vi "PressureGauge.vi"(4 "Error In":errorcluster, 7 "Command":string) -> (0 "Error Out":errorcluster, 3 "Response":string)   [LabVIEW 2018]
uses:
  MOKO_LabViewLibrary/MokoLowLevel/MokoLowLovelControl/MLLC_Mode.ctl
  data/PressureGaugeInfo.ctl
panel:
  in  "PRESSURESTORE":string="PRESSURESTORE"
  in  "Error Code":i32=5475
  in  "UtilitySettings":T2={"Permanent data"={"Информация об образце"={"Тип"="Манометр", "Владелец"="Компания \"MOKO\"", "Номер клейма"="111222", "Пределы допускаемой погрешности "=0.05, "Производственный № прибора"="111222333", "Наименование СИ"="Манометр"}, "Информация о поверке"={"Место проведения поверки"="Планета земля", "Поверку провел"="Johnny Respect", "Номер заказа"="1", "Номер рабочего места"="1", "ДД"=21.0, "ММ"="Январь", "ГГГГ"=2022.0, "№ протокола"="G-111111", "№ манометра"=5555.0}, "Характеристики манометра"={"Максимум шкалы"=10.0, "1-ая точка"=2.0, "Единица измерения"="МПа", "Цена деления"=2.0, "Класс точности"="0,4", "Минимум шкалы"=2.0, "Количество точек"=0.0}, "Условия поверки"={"Температура воздуха"=22.0, "Влажность воздуха"=60.0, "Давление"=750.0}, "Драйвер"="Simulation", "Поверяемая точка"=0.0}, "Saved Data"=variant(cluster{"Информация об образце":cluster{"Тип":string, "Владелец":string, "Номер клейма":string, "Пределы допускаемой погрешности ":dbl, "Производственный № прибора":string, "Наименование СИ":string}, "Информация о поверке":cluster{"Место проведения поверки":string, "Поверку провел":string, "Номер заказа":string, "Номер рабочего места":string, "ДД":dbl, "ММ":string, "ГГГГ":dbl, "№ протокола":string, "№ манометра":dbl}, "Характеристики манометра":cluster{"Максимум шкалы":dbl, "1-ая точка":dbl, "Единица измерения":string, "Цена деления":dbl, "Класс точности":string, "Минимум шкалы":dbl, "Количество точек":dbl}, "Условия поверки":cluster{"Температура воздуха":dbl, "Влажность воздуха":dbl, "Давление":dbl}, "Драйвер":string, "Поверяемая точка":dbl} {"Информация об образце"={"Тип"="Манометр", "Владелец"="Компания \"MOKO\"", "Номер клейма"="111222333", "Пределы допускаемой погрешности "=0.05, "Производственный № прибора"="111222333", "Наименование СИ"="Манометр"}, "Информация о поверке"={"Место проведения поверки"="Планета земля", "Поверку провел"="Johnny Respect", "Номер заказа"="1", "Номер рабочего места"="1", "ДД"=21.0, "ММ"="Январь", "ГГГГ"=2022.0, "№ протокола"="G-111111", "№ манометра"=1123123.0}, "Характеристики манометра"={"Максимум шкалы"=10.0, "1-ая точка"=2.0, "Единица измерения"="МПа", "Цена деления"=2.0, "Класс точности"="0,4", "Минимум шкалы"=2.0, "Количество точек"=0.0}, "Условия поверки"={"Температура воздуха"=22.0, "Влажность воздуха"=60.0, "Давление"=750.0}, "Драйвер"="Simulation", "Поверяемая точка"=0.0}), "waittime"=30000.0, "BAD"=0.0, "Defect"=FALSE}
  in  "Mode":T3=enum."Check"
  # "PressureGauge"
  # "Default Settings"
  # "Temporary data"
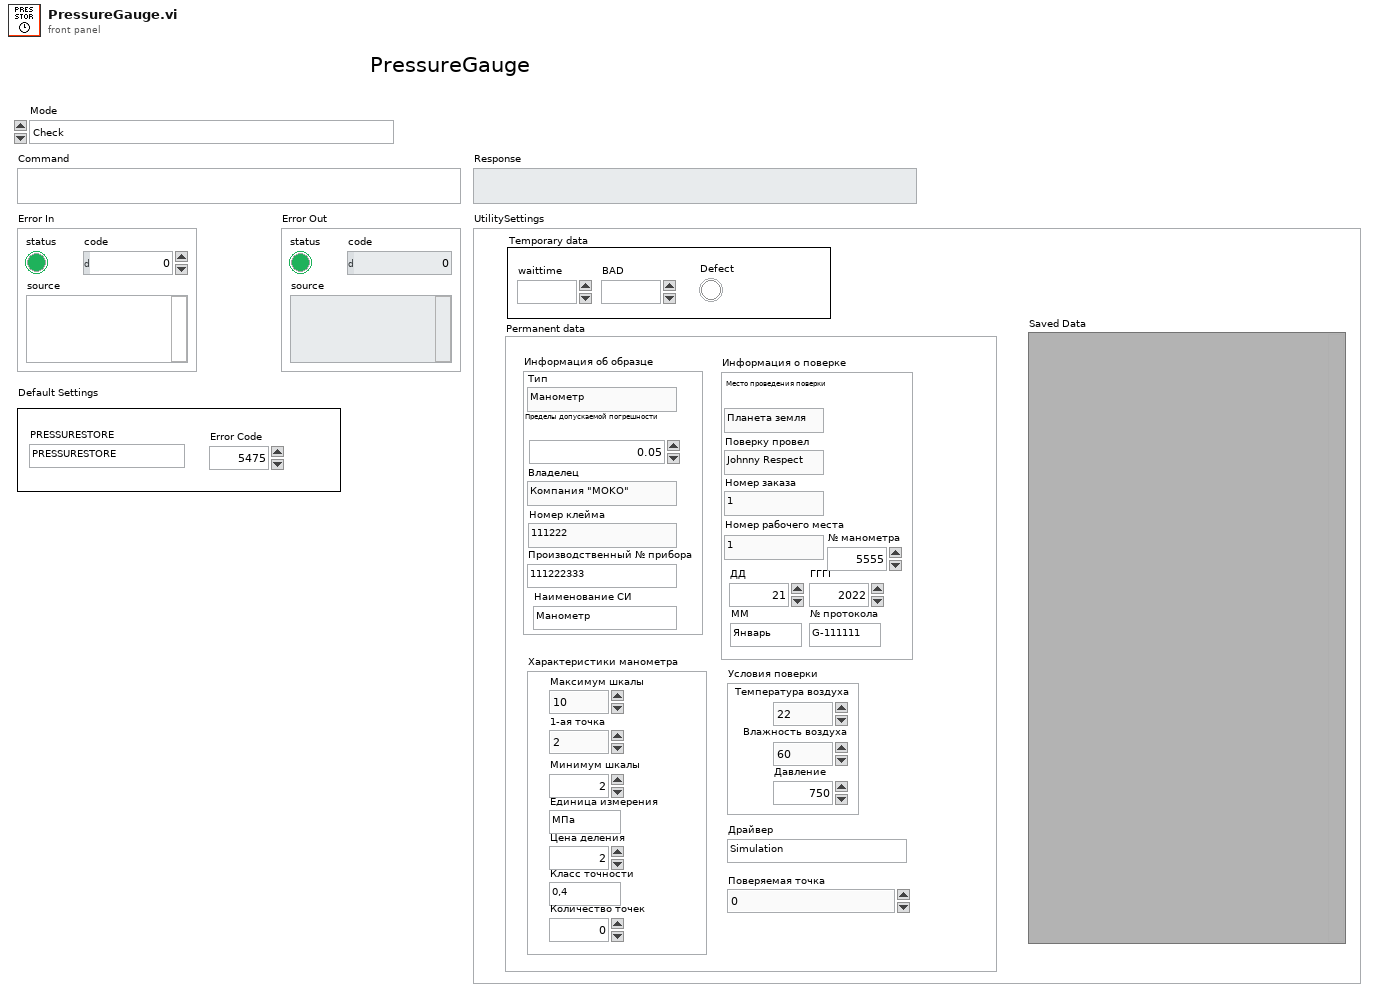
[diagram p1: front panel]
types:
  T1 = typedef "PressureGaugeInfo.ctl" = cluster{"Информация об образце":cluster{"Тип":string, "Владелец":string, "Номер клейма":string, "Пределы допускаемой погрешности ":dbl, "Производственный № прибора":string, "Наименование СИ":string}, "Информация о поверке":cluster{"Место проведения поверки":string, "Поверку провел":string, "Номер заказа":string, "Номер рабочего места":string, "ДД":dbl, "ММ":string, "ГГГГ":dbl, "№ протокола":string, "№ манометра":dbl}, "Характеристики манометра":cluster{"Максимум шкалы":dbl, "1-ая точка":dbl, "Единица измерения":string, "Цена деления":dbl, "Класс точности":string, "Минимум шкалы":dbl, "Количество точек":dbl}, "Условия поверки":cluster{"Температура воздуха":dbl, "Влажность воздуха":dbl, "Давление":dbl}, "Драйвер":string, "Поверяемая точка":dbl}
  T2 = cluster{"Permanent data":T1, "Saved Data":variant, "waittime":dbl, "BAD":dbl, "Defect":bool}
  T3 = typedef "MLLC_Mode.ctl" = enum16{"get", "set", "close", "Init", "Check"}
  T4 = typedef "MLLC_Error.ctl" = errorcluster
  T5 = typedef "MLLC_Command.ctl" = string
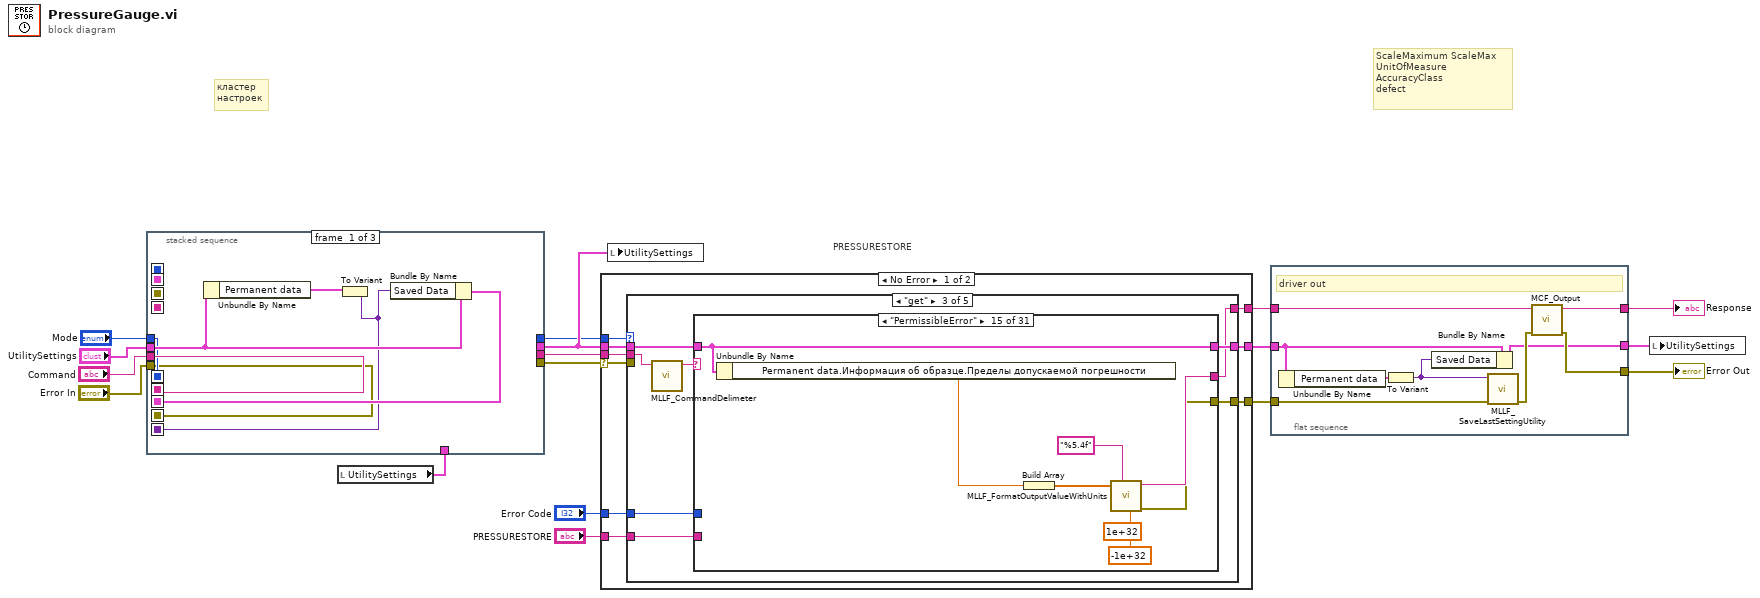
[diagram p0: block diagram]
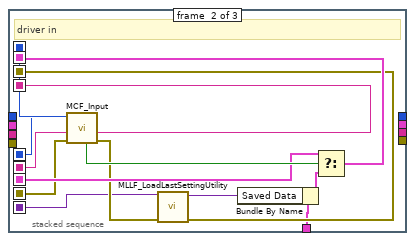
[diagram p2: hidden frame]
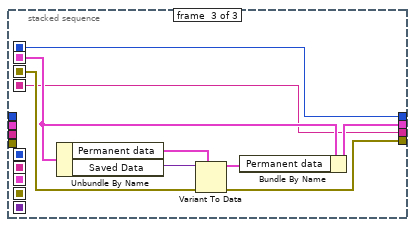
[diagram p3: hidden frame]
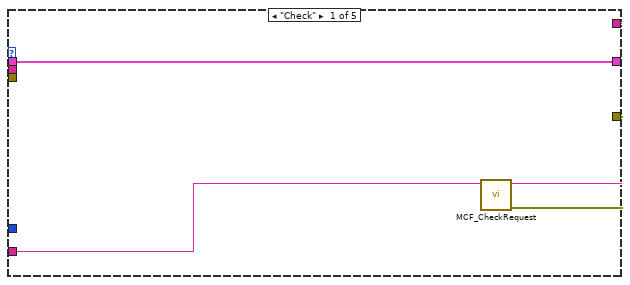
[diagram p4: hidden frame]
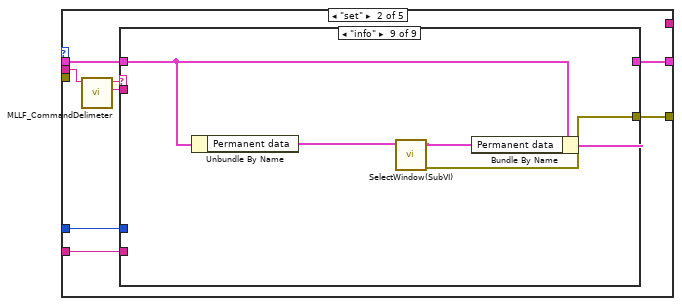
[diagram p5: hidden frame]
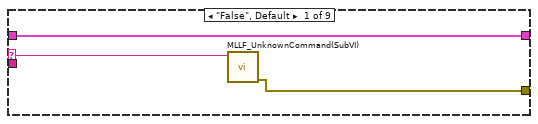
[diagram p6: hidden frame]
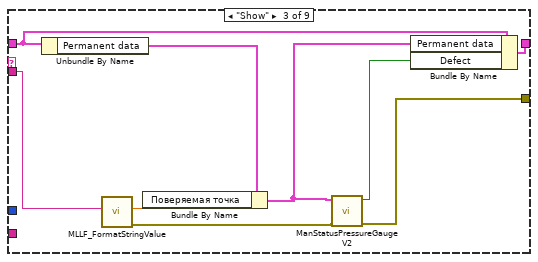
[diagram p8: hidden frame]
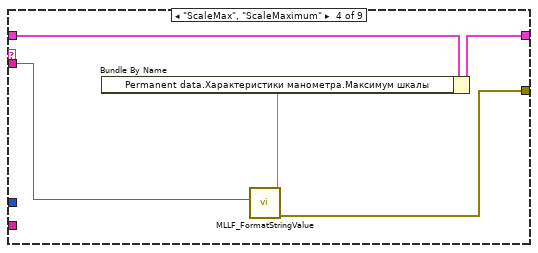
[diagram p9: hidden frame]
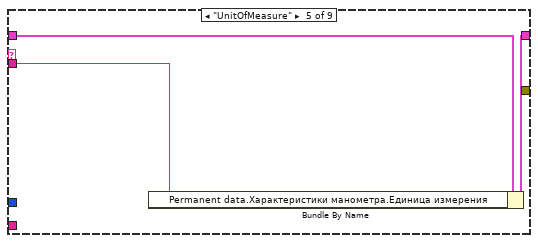
[diagram p10: hidden frame]
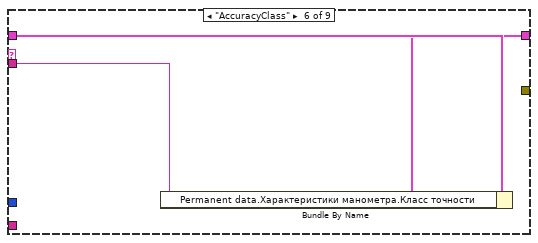
[diagram p11: hidden frame]
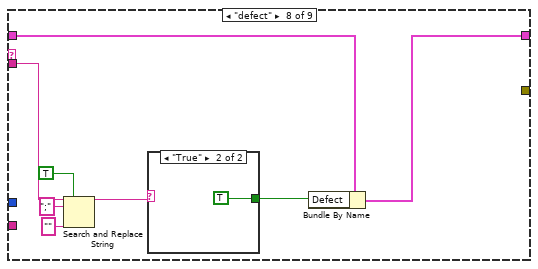
[diagram p13: hidden frame]
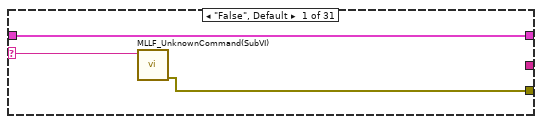
[diagram p15: hidden frame]
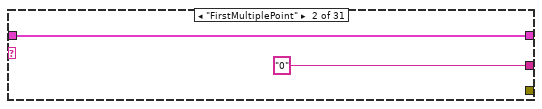
[diagram p16: hidden frame]
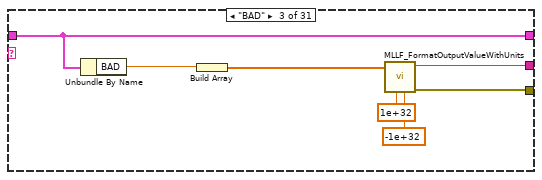
[diagram p17: hidden frame]
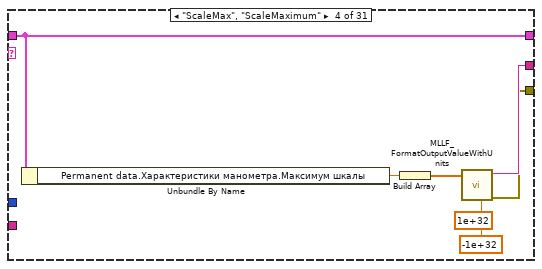
[diagram p18: hidden frame]
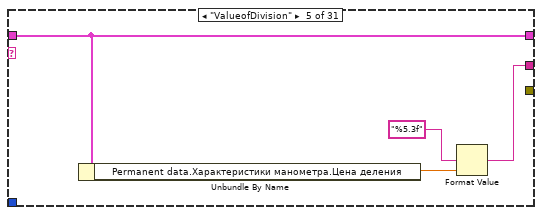
[diagram p19: hidden frame]
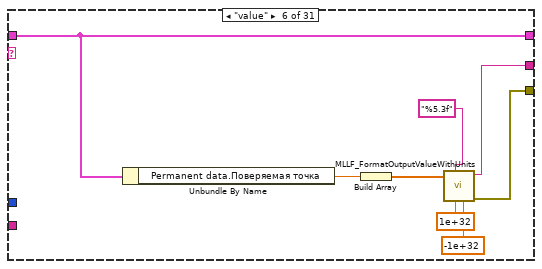
[diagram p20: hidden frame]
diagram:
  # "ScaleMaximum ScaleMax\nUnitOfMeasure\nAccuracyClass\ndefect"
  # "кластер\nнастроек"
  # "PRESSURESTORE"
  n1 = local read "UtilitySettings"() -> (w12:T2)
  n2 = stacked-sequence {
    seq-local: [w20 _ _] -> [_ w36 _]
    seq-local: [w19 _ _] -> [_ w37 _]
    seq-local: [w22 _ _] -> [_ w32 _]
    seq-local: [w18 _ _] -> [_ w31 _]
    seq-local: [w21 _ _] -> [_ w26 _]
    seq-local: [_ w27 _] -> [_ _ w43]
    seq-local: [_ w38 _] -> [_ _ w40]
    seq-local: [_ w35 _] -> [_ _ w39]
    seq-local: [_ w34 _] -> [_ _ w44]
    tunnel: "Command" -> [w20 _ _]
    tunnel: "Mode" -> [w19 _ _]
    tunnel: "Error In" -> [w18 _ _]
    tunnel: "UtilitySettings" -> [w23 _ _]
    tunnel: w12 -> [_ w25 _]
    tunnel: [_ _ w39] -> w8
    tunnel: [_ _ w42] -> w11
    tunnel: [_ _ w41] -> w10
    tunnel: [_ _ w40] -> w9
    frame #0 {
      n3 = Unbundle By Name(w23) -> ("Permanent data"=w24:T1)
      n4 = To Variant(anything=w24) -> (Variant=w21:variant)
      n5 = Bundle By Name(cluster=w23, "Saved Data"=w21) -> (w22:T2)
    }
    frame #1 {
      # "driver in"
      n6 = call "MCF_Input.vi"("Error In"=w31, "Command in"=w36, "Mode in"=w37) -> ("Error Out"=w30:errorcluster, "Command out"=w35:string, "Mode out"=w38:T3, "Boolean"=w33:bool)  [unwired: 5 in]
      n7 = call "MLLF_LoadLastSettingUtility.vi"("Error In"=w30, "Save data in"=w26) -> ("Error Out"=w27:errorcluster, "Save data out"=w29:variant)  [unwired: 8 in]
      n8 = Bundle By Name(cluster=w25, "Saved Data"=w29) -> (w28:T2)
      n9 = Select(t=w32, s=w33, f=w28) -> (s? t:f=w34:T2)
    }
    frame #2 {
      n10 = Unbundle By Name(w44) -> ("Permanent data"=w45:T1, "Saved Data"=w47:variant)
      n11 = Variant To Data(error in=w43, type=w45, Variant=w47) -> (data=w46:T1, error out=w41:errorcluster)
      n12 = Bundle By Name(cluster=w44, "Permanent data"=w46) -> (w42:T2)
    }
  }
  n13 = case shown="No Error" w10 {
    selector: w10 -> [w52 w233]
    tunnel: [w54 w233] -> w16
    tunnel: w9 -> [w56 _]
    tunnel: [w55 _] -> w14
    tunnel: w8 -> [w53 _]
    tunnel: w11 -> [w49 w232]
    tunnel: "Error Code" -> [w51 _]
    tunnel: "PRESSURESTORE" -> [w50 _]
    tunnel: [w48 w232] -> w15
    frame No Error {
      n14 = case shown="\"get\"" w56 {
        tunnel: [w58 _ w108 _ _] -> w55
        tunnel: [w57 w62 w109 _ _] -> w54
        tunnel: w53 -> [_ w68 w115 _ _]
        tunnel: w52 -> [_ _ _ _ _]
        tunnel: w51 -> [_ w67 w112 _ _]
        tunnel: w50 -> [w59 w64 w111 _ _]
        tunnel: w49 -> [w60 w66 w114 _ _]
        tunnel: [w60 w65 w113 _ _] -> w48
        frame "Check" {
          n15 = call "MCF_CheckRequest.vi"("Driver Name"=w59) -> ("Error Out"=w57:errorcluster, "Output String"=w58:string)  [unwired: 9 in]
        }
        frame "set" {
          n16 = call "MLLF_CommandDelimeter.vi"("command with param"=w68) -> ("param 1"=w61:string, "command"=w63:string)  [unwired: 6 in, 3 out]
          n17 = case shown="\"info\"" w63 {
            selector: w63 -> [w70 _ _ _ _ _ _ _ _]
            tunnel: w61 -> [_ _ w78 w82 w88 w92 _ w99 _]
            tunnel: [w69 _ w75 w86 _ _ _ _ w103] -> w62
            tunnel: w67 -> [_ _ _ _ _ _ _ _ _]
            tunnel: w66 -> [w71 w72 w80 w84 w89 w91 w93 w101 w107]
            tunnel: [w71 w72 w79 w83 w87 w90 w93 w100 w106] -> w65
            tunnel: w64 -> [_ _ _ _ _ _ _ _ _]
            frame "False", Default {
              n18 = call "MLLF_UnknownCommand(SubVI).vi"("Unknown command"=w70) -> ("error out"=w69:errorcluster)  [unwired: 10 in]
            }
            frame "<----MAIN FUNCTIONS---->" {
            }
            frame "Show" {
              n19 = Unbundle By Name(w80) -> ("Permanent data"=w74:T1)
              n20 = call "MLLF_FormatStringValue.vi"("String Value"=w78) -> ("error out"=w77:T4, "number"=w81:dbl)  [unwired: 8 in, 1 out]
              n21 = Bundle By Name(cluster=w74, "Поверяемая точка"=w81) -> (w73:T1)
              n22 = call "ManStatusPressureGaugeV2.vi"("Error In"=w77, "Show in"=w73) -> ("Error Out"=w75:errorcluster, "defect"=w76:bool)  [unwired: 8 in]
              n23 = Bundle By Name(cluster=w80, "Permanent data"=w73, "Defect"=w76) -> (w79:T2)
            }
            frame "ScaleMax", "ScaleMaximum" {
              n24 = call "MLLF_FormatStringValue.vi"("String Value"=w82) -> ("error out"=w86:T4, "number"=w85:dbl)  [unwired: 8 in, 1 out]
              n25 = Bundle By Name(cluster=w84, "Permanent data.Характеристики манометра.Максимум шкалы"=w85) -> (w83:T2)
            }
            frame "UnitOfMeasure" {
              n26 = Bundle By Name(cluster=w89, "Permanent data.Характеристики манометра.Единица измерения"=w88) -> (w87:T2)
            }
            frame "AccuracyClass" {
              n27 = Bundle By Name(cluster=w91, "Permanent data.Характеристики манометра.Класс точности"=w92) -> (w90:T2)
            }
            frame "---------ADDITIONAL---------" {
            }
            frame "defect" {
              n28 = Search and Replace String(replace all?=TRUE ("replace all? (F)"), input string=w99, search string=";", replace string="" ("replace string (\"\")")) -> (result string=w95:string)  [unwired: 4 in, 3 out]
              n29 = case shown="\"True\"" w95 {
                tunnel: [_ TRUE] -> w94
                frame "False", Default {
                }
                frame "True" {
                }
              }
              n30 = Bundle By Name(cluster=w101, "Defect"=w94) -> (w100:T2)
            }
            frame "info" {
              n31 = Unbundle By Name(w107) -> ("Permanent data"=w105:T1)
              n32 = call "SelectWindow(SubVI).vi"("Permanent data"=w105) -> ("Error Out"=w103:errorcluster, "Manometr out"=w104:T1)  [unwired: 9 in]
              n33 = Bundle By Name(cluster=w107, "Permanent data"=w104) -> (w106:T2)
            }
          }
        }
        frame "get" {
          n34 = call "MLLF_CommandDelimeter.vi"("command with param"=w115) -> ("command"=w110:string)  [unwired: 6 in, 4 out]
          n35 = case shown="\"PermissibleError\"" w110 {
            selector: w110 -> [w117 _ _ _ _ _ _ _ _ _ _ _ _ _ _ _ _ _ _ _ _ _ _ _ _ _ _ _ _ _ _]
            tunnel: [w116 _ w121 w128 _ w139 w148 _ _ w158 w164 _ _ _ w176 _ _ _ _ _ _ _ _ _ _ _ _ _ _ _ _] -> w109
            tunnel: w112 -> [_ _ _ _ _ _ _ _ _ _ _ _ _ _ _ _ _ _ _ _ _ _ _ _ _ _ _ _ _ _ _]
            tunnel: [w118 w120 w127 w133 w137 w145 w152 w154 w156 w162 w169 w171 w173 w175 w182 w183 w187 w188 w192 w194 w198 w199 w204 w205 w210 w212 w216 w220 w224 w226 w231] -> w113
            tunnel: w114 -> [w118 w120 w127 w133 w137 w145 w152 w154 w156 w162 w169 w171 w173 w175 w182 w183 w187 w188 w192 w194 w198 w199 w204 w205 w210 w212 w216 w220 w224 w226 w231]
            tunnel: w111 -> [_ _ _ _ _ _ _ _ _ _ _ _ _ _ _ _ _ _ _ _ _ _ _ _ _ _ _ _ _ _ _]
            tunnel: [_ "0" ("string") w122 w129 w134 w140 w147 w153 w155 w157 w165 w170 w172 w174 w178 w184 w185 w189 w190 w193 w195 w200 w201 w206 w207 w211 w213 w217 w221 w225 w227] -> w108
            frame "False", Default {
              n36 = call "MLLF_UnknownCommand(SubVI).vi"("Unknown command"=w117) -> ("error out"=w116:errorcluster)  [unwired: 10 in]
            }
            frame "FirstMultiplePoint" {
            }
            frame "BAD" {
              n37 = Unbundle By Name(w127) -> ("BAD"=w126:dbl)
              n38 = Build Array(w126) -> (w123:dbl[])
              n39 = call "MLLF_FormatOutputValueWithUnits.vi"("Lower limit"=-1e+32, "Upper limit"=1e+32, "ValuesIn"=w123) -> ("error out"=w121:T4, "Result string"=w122:T5)  [unwired: 7 in]
            }
            frame "ScaleMax", "ScaleMaximum" {
              (unwired) 1e+32 ("Upper limit")
              n40 = Unbundle By Name(w133) -> ("Permanent data.Характеристики манометра.Максимум шкалы"=w132:dbl)
              n41 = Build Array(w132) -> (w130:dbl[])
              n42 = call "MLLF_FormatOutputValueWithUnits.vi"("Lower limit"=-1e+32, "ValuesIn"=w130) -> ("error out"=w128:T4, "Result string"=w129:T5)  [unwired: 8 in]
            }
            frame "ValueofDivision" {
              n43 = Unbundle By Name(w137) -> ("Permanent data.Характеристики манометра.Цена деления"=w135:dbl)
              n44 = Format Value(format string="%5.3f", value (0)=w135) -> (output string=w134:string)  [unwired: 1 in]
            }
            frame "value" {
              n45 = Unbundle By Name(w145) -> ("Permanent data.Поверяемая точка"=w144:dbl)
              n46 = Build Array(w144) -> (w141:dbl[])
              n47 = call "MLLF_FormatOutputValueWithUnits.vi"("Lower limit"=-1e+32, "Upper limit"=1e+32, "Format"="%5.3f" ("format string"), "ValuesIn"=w141) -> ("error out"=w139:T4, "Result string"=w140:T5)  [unwired: 6 in]
            }
            frame "FirstDigitizedPoint", "FirstPoint" {
              (unwired) 1e+32 ("Upper limit")
              n48 = Unbundle By Name(w152) -> ("Permanent data.Характеристики манометра.1-ая точка"=w151:dbl)
              n49 = Build Array(w151) -> (w149:dbl[])
              n50 = call "MLLF_FormatOutputValueWithUnits.vi"("Lower limit"=-1e+32, "Format"="%5.3f" ("format string"), "ValuesIn"=w149) -> ("error out"=w148:T4, "Result string"=w147:T5)  [unwired: 7 in]
            }
            frame "SerialNumberDevice" {
              n51 = Unbundle By Name(w154) -> ("Permanent data.Информация об образце.Производственный № прибора"=w153:string)
            }
            frame "NameMI" {
              n52 = Unbundle By Name(w156) -> ("Permanent data.Информация об образце.Наименование СИ"=w155:string)
            }
            frame "NumOfPoints" {
              (unwired) 1e+32 ("Upper limit")
              n53 = Unbundle By Name(w162) -> ("Permanent data.Характеристики манометра.Количество точек"=w161:dbl)
              n54 = Build Array(w161) -> (w159:dbl[])
              n55 = call "MLLF_FormatOutputValueWithUnits.vi"("Lower limit"=-1e+32, "ValuesIn"=w159) -> ("error out"=w158:T4, "Result string"=w157:T5)  [unwired: 8 in]
            }
            frame "ScaleMin" {
              (unwired) 1e+32 ("Upper limit")
              n56 = Unbundle By Name(w169) -> ("Permanent data.Характеристики манометра.Минимум шкалы"=w168:dbl)
              n57 = Build Array(w168) -> (w166:dbl[])
              n58 = call "MLLF_FormatOutputValueWithUnits.vi"("Lower limit"=-1e+32, "Format"="%5.3f" ("format string"), "ValuesIn"=w166) -> ("error out"=w164:T4, "Result string"=w165:T5)  [unwired: 7 in]
            }
            frame "UnitOfMeasure" {
              n59 = Unbundle By Name(w171) -> ("Permanent data.Характеристики манометра.Единица измерения"=w170:string)
            }
            frame "AccuracyClass" {
              n60 = Unbundle By Name(w173) -> ("Permanent data.Характеристики манометра.Класс точности"=w172:string)
            }
            frame "TypeofUnit" {
              n61 = Unbundle By Name(w175) -> ("Permanent data.Информация об образце.Тип"=w174:string)
            }
            frame "PermissibleError" {
              (unwired) 1e+32 ("Upper limit")
              n62 = Unbundle By Name(w182) -> ("Permanent data.Информация об образце.Пределы допускаемой погрешности"=w181:dbl)
              n63 = Build Array(w181) -> (w179:dbl[])
              n64 = call "MLLF_FormatOutputValueWithUnits.vi"("Lower limit"=-1e+32, "Format"="%5.4f" ("format string"), "ValuesIn"=w179) -> ("error out"=w176:T4, "Result string"=w178:T5)  [unwired: 7 in]
            }
            frame "StampNumber" {
              n65 = Unbundle By Name(w183) -> ("Permanent data.Информация об образце.Номер клейма"=w184:string)
            }
            frame "Owner" {
              n66 = Unbundle By Name(w187) -> ("Permanent data.Информация об образце.Владелец"=w186:string)
              n67 = call "MLLF_ReplaceTwoQuotesWithOne.vi"("String in"=w186) -> ("Result string"=w185:string)  [unwired: 7 in, 3 out]
            }
            frame "Verifier" {
              n68 = Unbundle By Name(w188) -> ("Permanent data.Информация о поверке.Поверку провел"=w189:string)
            }
            frame "VerificationLocation" {
              n69 = Unbundle By Name(w192) -> ("Permanent data.Информация о поверке.Место проведения поверки"=w191:string)
              n70 = call "MLLF_ReplaceTwoQuotesWithOne.vi"("String in"=w191) -> ("Result string"=w190:string)  [unwired: 7 in, 3 out]
            }
            frame "WorkplaceNumber" {
              n71 = Unbundle By Name(w194) -> ("Permanent data.Информация о поверке.Номер рабочего места"=w193:string)
            }
            frame "UnitNumber" {
              n72 = Unbundle By Name(w198) -> ("Permanent data.Информация о поверке.№ манометра"=w196:dbl)
              n73 = Format Value(format string="%5.1f", value (0)=w196) -> (output string=w195:string)  [unwired: 1 in]
            }
            frame "OrderNumber" {
              n74 = Unbundle By Name(w199) -> ("Permanent data.Информация о поверке.Номер заказа"=w200:string)
            }
            frame "Day" {
              n75 = Unbundle By Name(w204) -> ("Permanent data.Информация о поверке.ДД"=w202:dbl)
              n76 = Format Value(format string="%#g", value (0)=w202) -> (output string=w201:string)  [unwired: 1 in]
            }
            frame "Month" {
              n77 = Unbundle By Name(w205) -> ("Permanent data.Информация о поверке.ММ"=w206:string)
            }
            frame "Year" {
              n78 = Unbundle By Name(w210) -> ("Permanent data.Информация о поверке.ГГГГ"=w208:dbl)
              n79 = Format Value(format string="%#g", value (0)=w208) -> (output string=w207:string)  [unwired: 1 in]
            }
            frame "ProtocolNumber" {
              n80 = Unbundle By Name(w212) -> ("Permanent data.Информация о поверке.№ протокола"=w211:string)
            }
            frame "Temperature" {
              n81 = Unbundle By Name(w216) -> ("Permanent data.Условия поверки.Температура воздуха"=w215:dbl)
              n82 = Format Value(format string="%5.1f", value (0)=w215) -> (output string=w213:string)  [unwired: 1 in]
            }
            frame "AmbientPressure" {
              n83 = Unbundle By Name(w220) -> ("Permanent data.Условия поверки.Давление"=w218:dbl)
              n84 = Format Value(format string="%5.1f", value (0)=w218) -> (output string=w217:string)  [unwired: 1 in]
            }
            frame "Humidity" {
              n85 = Unbundle By Name(w224) -> ("Permanent data.Условия поверки.Влажность воздуха"=w222:dbl)
              n86 = Format Value(format string="%5.1f", value (0)=w222) -> (output string=w221:string)  [unwired: 1 in]
            }
            frame "Driver" {
              n87 = Unbundle By Name(w226) -> ("Permanent data.Драйвер"=w225:string)
            }
            frame "defect" {
              n88 = Unbundle By Name(w231) -> ("Defect"=w228:bool)
              n89 = Select(t="True" ("string"), s=w228, f="False" ("string")) -> (s? t:f=w227:string)
            }
          }
        }
        frame "close" {
        }
        frame "Init" {
        }
      }
    }
    frame Error {
    }
  }
  n90 = local write "UtilitySettings"(w11) -> ()
  n91 = flat-sequence {
    tunnel: [w242] -> w6
    tunnel: [w241] -> w4
    tunnel: w14 -> [w240]
    tunnel: w16 -> [w239]
    tunnel: w15 -> [w235]
    tunnel: [w237] -> w13
    frame #0 {
      # "driver out"
      n92 = Unbundle By Name(w235) -> ("Permanent data"=w234:T1)
      n93 = To Variant(anything=w234) -> (Variant=w236:variant)
      n94 = Bundle By Name(cluster=w235, "Saved Data"=w236) -> (w237:T2)
      n95 = call "MLLF_SaveLastSettingUtility.vi"("error in"=w239, "Saved Data"=w236) -> ("error out"=w238:T4)  [unwired: 8 in, 1 out]
      n96 = call "MCF_Output.vi"("Error In"=w238, "Input"=w240) -> ("Error Out"=w241:errorcluster, "Output"=w242:string)  [unwired: 8 in]
    }
  }
  n97 = local write "UtilitySettings"(w13) -> ()
  "Response" <- w6
  "Error Out" <- w4
